vi "Save Subject Params.vi"(4 "Subject Parameters":T1={"Subject"=1, "Left GPD Params"={"% Cycle Delay"=0.0, "Min % Cycle LR to ISw "=0.0, "Min % Cycle LR to MSw"=0.0, "Min % Cycle LR to TSw"=0.0, "Max % Cycle ISw to MSw"=0.0, "Min % Cycle TSw to LR"=0.0, "Max % Cycle TSw to LR"=0.0, "LR Min Gyro Z Threshold"=0.0, "LR Min Gyro Z Width"=0.0, "ISw Peak Threshold"=0.0, "ISw Peak Width"=0.0, "TSw Valley Threshold"=0.0, "TSw Valley Width (ms)"=0.0, "Max Cycle Time (s)"=0.0, "Mean Computation Window"=0.0, "CP subject?"=FALSE}, "Right GPD Params"={"% Cycle Delay"=0.0, "Min % Cycle LR to ISw "=0.0, "Min % Cycle LR to MSw"=0.0, "Min % Cycle LR to TSw"=0.0, "Max % Cycle ISw to MSw"=0.0, "Min % Cycle TSw to LR"=0.0, "Max % Cycle TSw to LR"=0.0, "LR Min Gyro Z Threshold"=0.0, "LR Min Gyro Z Width"=0.0, "ISw Peak Threshold"=0.0, "ISw Peak Width"=0.0, "TSw Valley Threshold"=0.0, "TSw Valley Width (ms)"=0.0, "Max Cycle Time (s)"=0.0, "Mean Computation Window"=0.0, "CP subject?"=FALSE}, "Left Stim Params"={"Stim Pattern Values"=[], "Pulse Duration"=[], "Current"=[]}, "Right Stim Params"={"Stim Pattern Values"=[], "Pulse Duration"=[], "Current"=[]}, "Left Train length"=[], "Right Train length"=[]} {"Subject" items=["Subject 0", "Subject 1", "Subject 2", "Subject 3", "Subject 4", "Subject 5", "Subject 6", "Subject 7", "Subject 8", "Subject 9", "Subject 10", "Subject 11", "Subject 12", "Subject 13", "Subject 14", "Subject 15", "Subject 16", "Subject 17", "Subject 18", "Subject 19", "Subject 20", "Subject 21", "Subject 22", "Subject 23", "Subject 24", "Subject 25", "Subject 26", "Subject 27", "Subject 28", "Subject 29", "Subject 30", "Subject 31", "Subject 32", "Subject 33", "Subject 34", "Subject 35", "Subject 36", "Subject 37", "Subject 38", "Subject 39", "Subject 40"]}, 5 "Subject Parameters File":path=path "Z:/Lee Lab/CP FES Walking 2018/Subject Parameters/subj_10_threshold_params.txt") -> (2 "Subject Parameters File":path=path "Z:/Lee Lab/CP FES Walking 2018/Subject Parameters/subj_10_threshold_params.txt")   [LabVIEW 2019]
uses:
  Controls/Subject Params.ctl
  Controls/Subject.ctl
  Controls/GPD Side Parameters.ctl
  Controls/Type Defs/Stim Parameters.ctl
  Controls/Stim off-half-ful.ctl
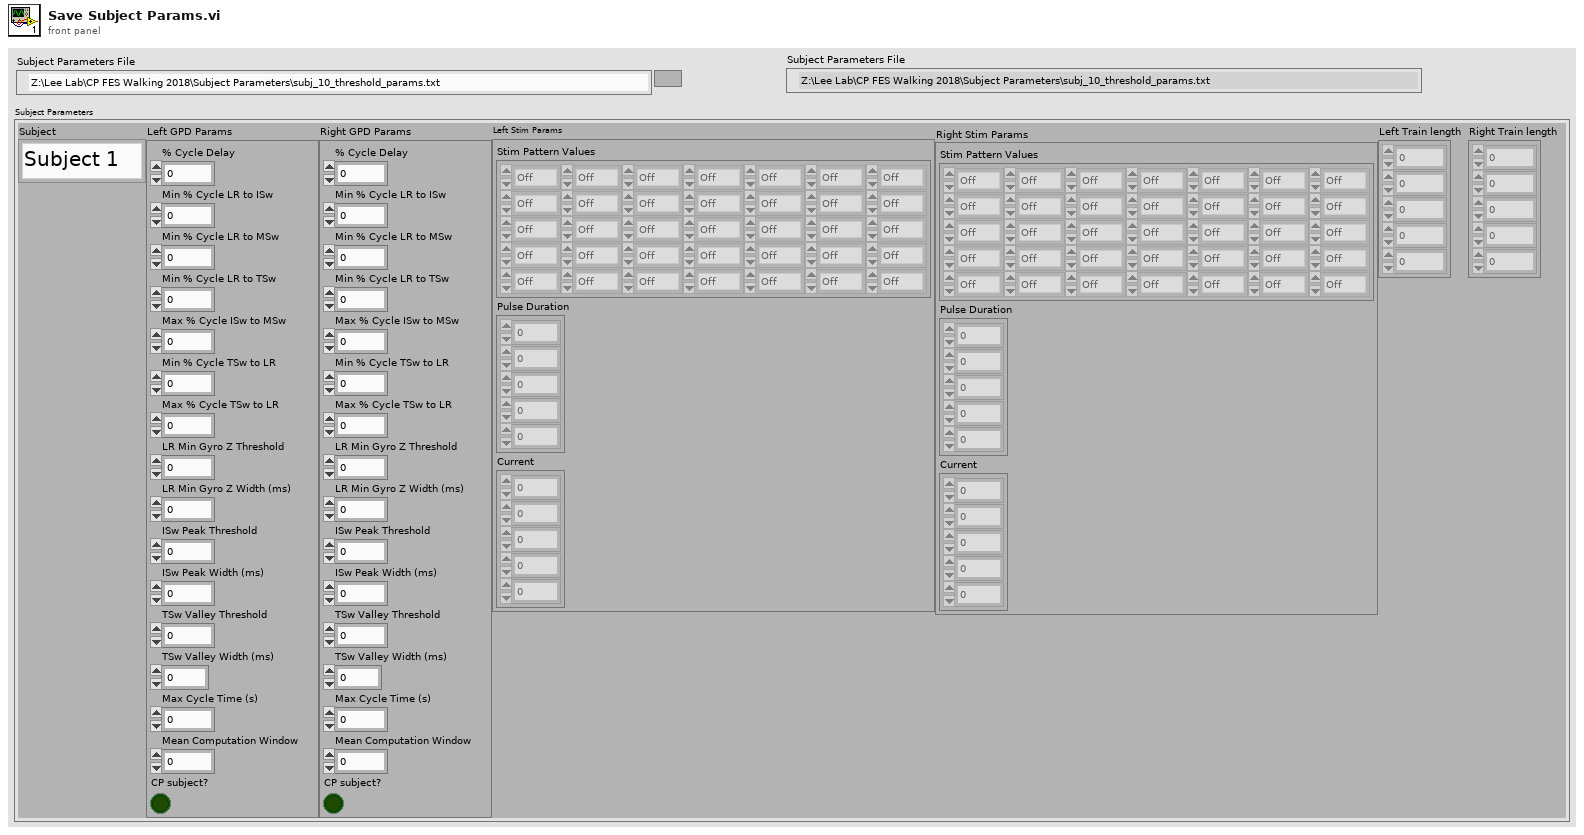
[diagram p1: front panel]
types:
  T1 = typedef "Subject Params.ctl" = cluster{"Subject":T2, "Left GPD Params":T3, "Right GPD Params":T3, "Left Stim Params":T4, "Right Stim Params":T4, "Left Train length":i64[], "Right Train length":i64[]}
  T2 = typedef "Subject.ctl" = u16
  T3 = typedef "GPD Side Parameters.ctl" = cluster{"% Cycle Delay":dbl, "Min % Cycle LR to ISw ":dbl, "Min % Cycle LR to MSw":dbl, "Min % Cycle LR to TSw":dbl, "Max % Cycle ISw to MSw":dbl, "Min % Cycle TSw to LR":dbl, "Max % Cycle TSw to LR":dbl, "LR Min Gyro Z Threshold":dbl, "LR Min Gyro Z Width":dbl, "ISw Peak Threshold":dbl, "ISw Peak Width":dbl, "TSw Valley Threshold":dbl, "TSw Valley Width (ms)":dbl, "Max Cycle Time (s)":dbl, "Mean Computation Window":dbl, "CP subject?":bool}
  T4 = typedef "Stim Parameters.ctl" = cluster{"Stim Pattern Values":T5[][], "Pulse Duration":i64[], "Current":i64[]}
  T5 = typedef "Stim off-half-ful.ctl" = enum16{"Off", "Half", "Full"}
  T6 = enum16{"open", "replace", "create", "open or create", "replace or create", "replace or create with confirmation"}
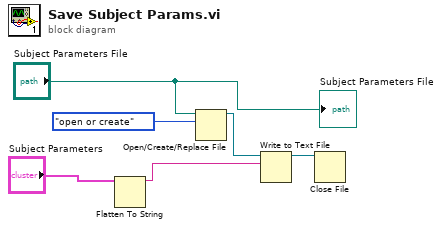
[diagram p0: block diagram]
diagram:
  n1 = Flatten To String(anything="Subject Parameters") -> (data string=w4:string)  [unwired: 3 in, 2 out]
  n2 = Open/Create/Replace File(file path (use dialog)="Subject Parameters File", operation (0:open)=T6."open or create") -> (refnum out=w5:refnum<file>)  [unwired: 4 in, 2 out]
  n3 = Write to Text File(file (use dialog)=w5, text=w4) -> (refnum out=w3:refnum<file>)  [unwired: 2 in, 2 out]
  n4 = Close File(refnum=w3) -> ()  [unwired: 1 in, 2 out]
  "Subject Parameters File" <- "Subject Parameters File"
